vi "main.vi"() -> ()   [LabVIEW 2023]
uses:
  #typdef_state.ctl
panel:
  in  "B":dbl
  in  "A":dbl
  out "Result":dbl
  in  "AbsoluteValue":bool
  in  "Divide":bool
  in  "Multiply":bool
  in  "Substract":bool
  in  "Add":bool
  in  "Exit":bool
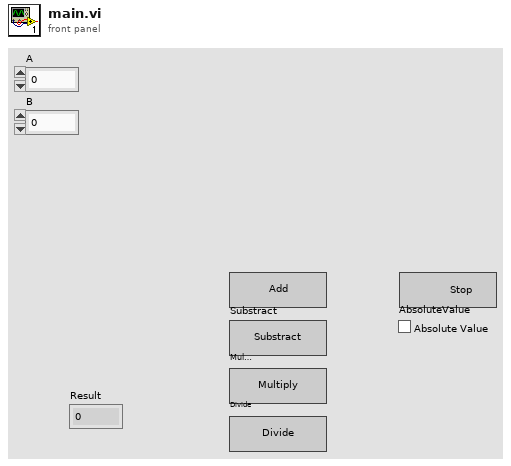
[diagram p1: front panel]
types:
  T1 = typedef "#typdef_state.ctl" = enum16{"Aplication Error", "Inicialization", "Idle", "Add", "Substract", "Multiply", "Divide", "AbsoluteValue", "Exit"}
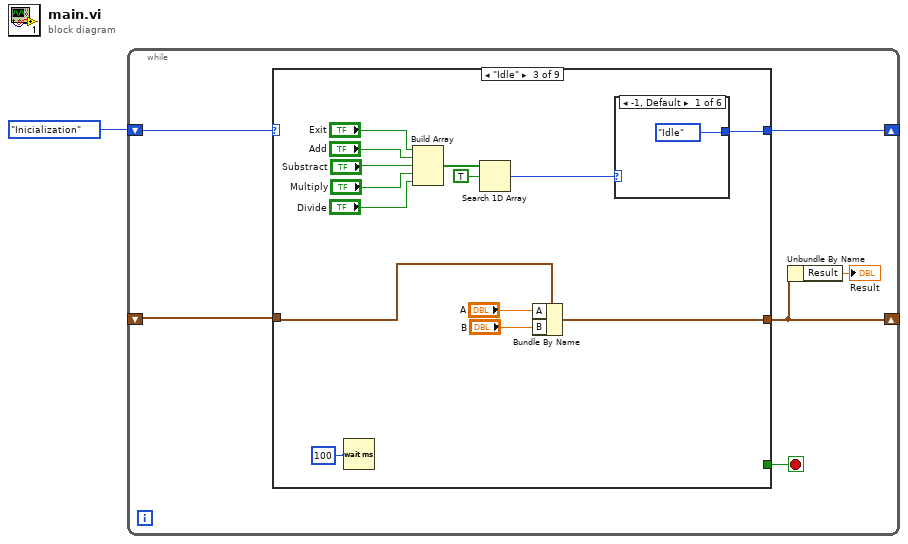
[diagram p0: block diagram]
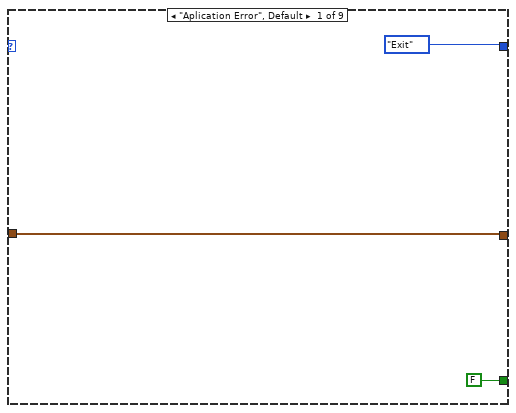
[diagram p2: hidden frame]
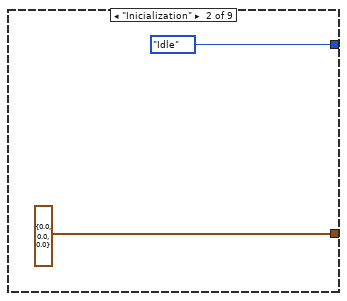
[diagram p3: hidden frame]
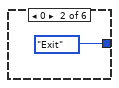
[diagram p4: hidden frame]
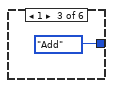
[diagram p5: hidden frame]
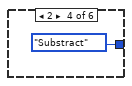
[diagram p6: hidden frame]
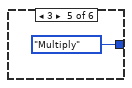
[diagram p7: hidden frame]
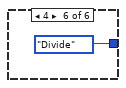
[diagram p8: hidden frame]
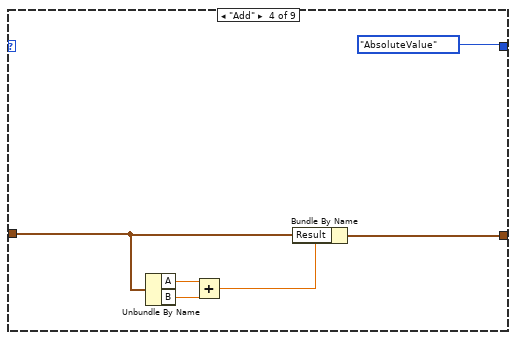
[diagram p9: hidden frame]
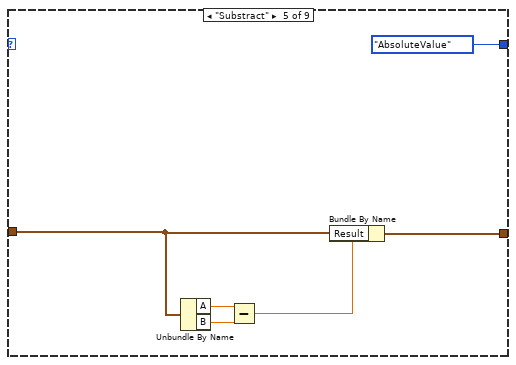
[diagram p10: hidden frame]
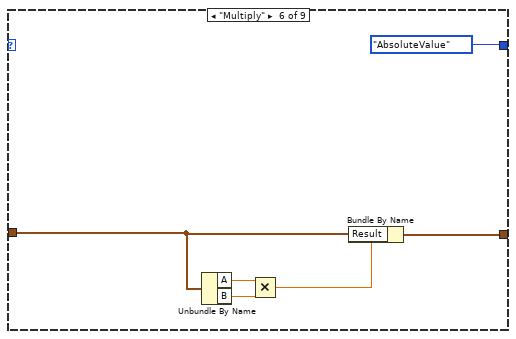
[diagram p11: hidden frame]
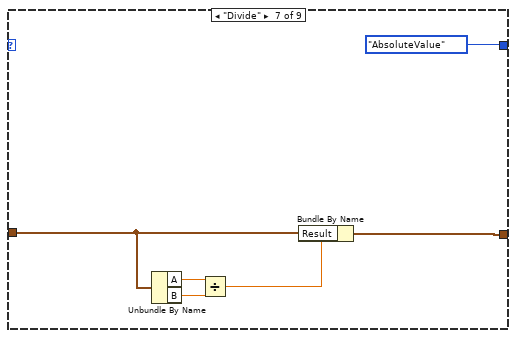
[diagram p12: hidden frame]
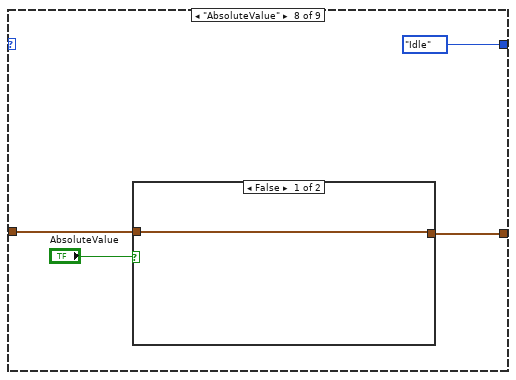
[diagram p13: hidden frame]
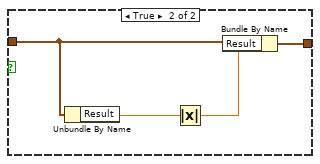
[diagram p14: hidden frame]
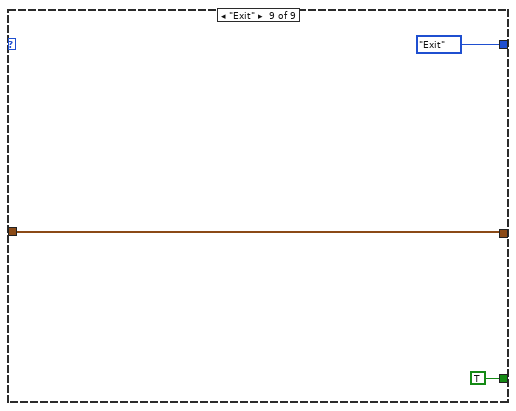
[diagram p15: hidden frame]
diagram:
  n1 = while {
    shift-right: [w6] -> _
    shift-left: #typdef_state."Inicialization" ("State") -> [w7]
    shift-right: [w3] -> _
    shift-left: _ -> [w5]
    stop <- w4 stop-if-true
    n2 = case shown="\"Idle\"" w7 {
      tunnel: [w10 cluster{"A":dbl, "B":dbl, "Result":dbl} {"A"=0.0, "B"=0.0, "Result"=0.0} ("DATA") w16 w33 w39 w45 w54 w58 w68] -> w3
      tunnel: [#typdef_state."Exit" ("State") #typdef_state."Idle" ("State") w17 #typdef_state."AbsoluteValue" ("State") #typdef_state."AbsoluteValue" ("State") #typdef_state."AbsoluteValue" ("State") #typdef_state."AbsoluteValue" ("State") #typdef_state."Idle" ("State") #typdef_state."Exit" ("State")] -> w6
      tunnel: w5 -> [w10 _ w15 w34 w40 w46 w55 w59 w68]
      tunnel: [FALSE _ _ _ _ _ _ _ TRUE] -> w4
      frame "Aplication Error", Default {
      }
      frame "Inicialization" {
      }
      frame "Idle" {
        n3 = Wait (ms)(milliseconds to wait=u32 100) -> ()  [unwired: 1 out]
        n4 = Build Array("Exit", "Add", "Substract", "Multiply", "Divide") -> (w20:bool[])
        n5 = Search 1D Array(1D array=w20, element=TRUE) -> (index of element=w18:i32)  [unwired: 1 in]
        n6 = Bundle By Name(cluster=w15, "A"="A", "B"="B") -> (w16:cluster{"A":dbl, "B":dbl, "Result":dbl})
        n7 = case shown="-1, Default" w18 {
          tunnel: [#typdef_state."Idle" ("State") #typdef_state."Exit" ("State") #typdef_state."Add" ("State") #typdef_state."Substract" ("State") #typdef_state."Multiply" ("State") #typdef_state."Divide" ("State")] -> w17
          frame -1, Default {
          }
          frame 0 {
          }
          frame 1 {
          }
          frame 2 {
          }
          frame 3 {
          }
          frame 4 {
          }
        }
      }
      frame "Add" {
        n8 = Unbundle By Name(w34) -> ("A"=w37:dbl, "B"=w36:dbl)
        n9 = Add(x=w37, y=w36) -> (x+y=w35:dbl)
        n10 = Bundle By Name(cluster=w34, "Result"=w35) -> (w33:cluster{"A":dbl, "B":dbl, "Result":dbl})
      }
      frame "Substract" {
        n11 = Unbundle By Name(w40) -> ("A"=w41:dbl, "B"=w42:dbl)
        n12 = Subtract(x=w41, y=w42) -> (x-y=w43:dbl)
        n13 = Bundle By Name(cluster=w40, "Result"=w43) -> (w39:cluster{"A":dbl, "B":dbl, "Result":dbl})
      }
      frame "Multiply" {
        n14 = Unbundle By Name(w46) -> ("A"=w47:dbl, "B"=w48:dbl)
        n15 = Multiply(x=w47, y=w48) -> (x*y=w49:dbl)
        n16 = Bundle By Name(cluster=w46, "Result"=w49) -> (w45:cluster{"A":dbl, "B":dbl, "Result":dbl})
      }
      frame "Divide" {
        n17 = Unbundle By Name(w55) -> ("A"=w53:dbl, "B"=w52:dbl)
        n18 = Divide(x=w53, y=w52) -> (x/y=w51:dbl)
        n19 = Bundle By Name(cluster=w55, "Result"=w51) -> (w54:cluster{"A":dbl, "B":dbl, "Result":dbl})
      }
      frame "AbsoluteValue" {
        n20 = case shown="False" "AbsoluteValue" {
          tunnel: w59 -> [w61 w65]
          tunnel: [w61 w64] -> w58
          frame False {
          }
          frame True {
            n21 = Unbundle By Name(w65) -> ("Result"=w63:dbl)
            n22 = Absolute Value(x=w63) -> (abs(x)=w62:dbl)
            n23 = Bundle By Name(cluster=w65, "Result"=w62) -> (w64:cluster{"A":dbl, "B":dbl, "Result":dbl})
          }
        }
      }
      frame "Exit" {
      }
    }
    n24 = Unbundle By Name(w3) -> ("Result"=→"Result":dbl)
  }
